vi "Actor Core.vi"(8 "error in":errorcluster, 11 "CS++DIM-Server in":refnum<class "CS++DIM-Server.lvclass">) -> (0 "error out":errorcluster, 3 "Actor out":refnum<class "Actor.lvclass">)   [LabVIEW 2015, in "CS++DIM-Server.lvlib" / "CS++DIM-Server.lvclass"]
doc: "(<B>Filename</B>: Actor Framework.lvlib:Actor.lvclass:Actor Core.vi)\n\nReceives messages to the actor, reacts to them, and initiates any error handling that may shut the actor down.\n\nDescendant classes may override this VI to append parallel tasks for the actor to complete while it handles messages. Overrides use the Call Parent Method node."
uses:
  CS++DIM-Server.lvclass
  <vilib>/ActorFramework/Actor/Actor.lvclass
  CSPP_Core/Actors/CS++BaseActor/CS++BaseActor.lvclass/CS++BaseActor.ctl
  CS++DIM-Server.lvclass/CS++DIM-Server.ctl
  <vilib>/ActorFramework/Actor/Actor.lvclass/Actor.ctl
  <vilib>/ActorFramework/Message Enqueuer/Message Enqueuer.lvclass/Message Enqueuer.ctl
  <vilib>/ActorFramework/Message Enqueuer/Init from Existing Queue.vi
  <vilib>/ActorFramework/Message Enqueuer/Enqueue.vi
  <vilib>/ActorFramework/Message Priority Queue/Priority Enqueue.vi
  <vilib>/ActorFramework/Stop Msg/Stop Msg.lvclass
  <vilib>/ActorFramework/Message Enqueuer/Message Enqueuer.lvclass
  CSPP_Core/Actors/CS++BaseActor/CS++BaseActor.lvclass
panel:
  out "Chart":dbl(graph)
  out "Update Rate":dbl[unit]
  out "Last Update":timestamp
  in  "Stop Button":bool
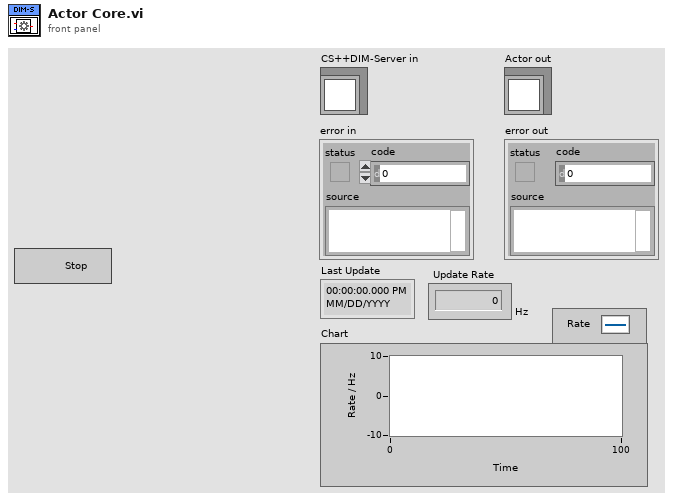
[diagram p1: front panel]
types:
  T1 = enum32{"Invalid", "Standard", "Closed", "Hidden", "Minimized", "Maximized"}
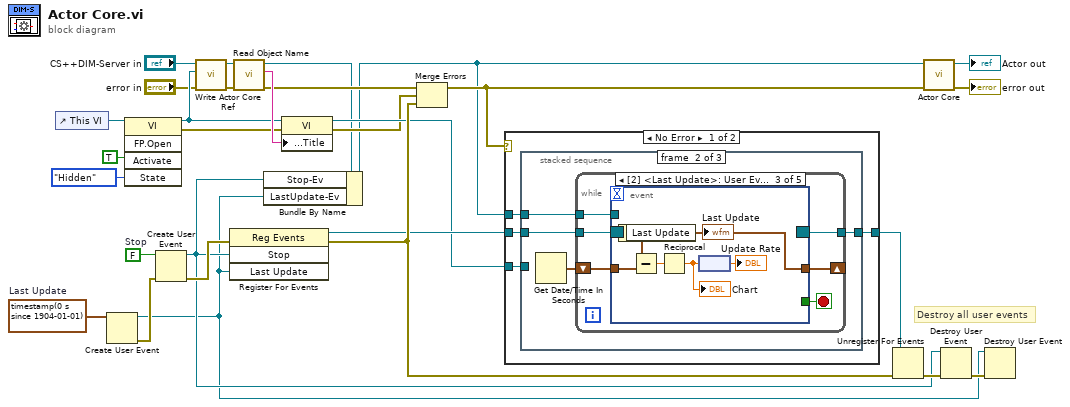
[diagram p0: block diagram]
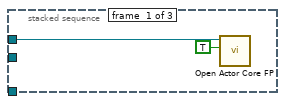
[diagram p2: hidden frame]
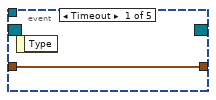
[diagram p3: hidden frame]
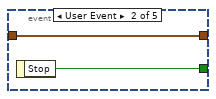
[diagram p4: hidden frame]
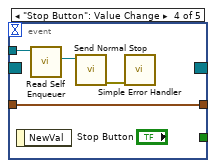
[diagram p5: hidden frame]
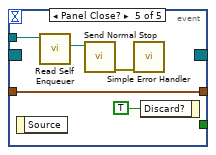
[diagram p6: hidden frame]
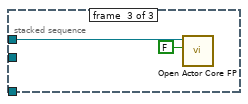
[diagram p7: hidden frame]
diagram:
  w7 = timestamp(0 s since 1904-01-01)  # Last Update
  w21 = FALSE  # Stop
  # "Destroy all user events"
  n1 = control-ref of="This VI"() -> (w25:refnum<vi>)
  n2 = Create User Event(user event datatype=w7) -> (user event=w1:refnum<user-event>, error out=w6:errorcluster)  [unwired: 1 in]
  n3 = invoke class="VI" method="FP.Open"(reference=w25, "Activate"=TRUE ("Activate?"), "State"=T1."Hidden") -> (reference out=w14:refnum<vi>, error out=w18:errorcluster)  [unwired: 2 in, 3 out]
  n4 = Create User Event(user event datatype=w21, error in=w6) -> (user event=w5:refnum<user-event>, error out=w19:errorcluster)
  n5 = call "Write Actor Core Ref.vi"("error in (no error)"="error in", "Actor Core Ref"=w14, "CS++BaseActor in"="CS++DIM-Server in") -> ("error out"=w17:errorcluster, "CS++BaseActor out"=w16:refnum<class "CS++DIM-Server.lvclass">)  [unwired: 7 in]
  n6 = register-events(error in=w19, w5, w1) -> (reference out=w28:refnum<event-registration>, error out=w29:errorcluster)  [unwired: 1 in]
  n7 = call "Read Object Name.vi"("error in (no error)"=w17, "CS++BaseActor in"=w16) -> ("error out"=w15:errorcluster, "Object Name"=w22:string, "CS++BaseActor out"=w4:refnum<class "CS++DIM-Server.lvclass">)  [unwired: 7 in]
  n8 = Bundle By Name(cluster=w4, "Stop-Ev"=w5, "LastUpdate-Ev"=w1) -> (w3:refnum<class "CS++DIM-Server.lvclass">)
  n9 = property class="VI"(reference=w14, error in=w18, "Front Panel.Title"=w22) -> (reference out=w27:refnum<vi>, error out=w20:errorcluster)
  n10 = Merge Errors(w15, w20, w29) -> (w26:errorcluster)
  n11 = case shown="No Error" w26 {
    tunnel: w3 -> [w33 _]
    tunnel: w28 -> [w32 w65]
    tunnel: [w31 w65] -> w10
    tunnel: w27 -> [w30 _]
    frame No Error {
      n12 = stacked-sequence {
        tunnel: w33 -> [w35 w38 w64]
        tunnel: w32 -> [_ w39 _]
        tunnel: [_ w37 _] -> w31
        tunnel: w30 -> [_ _ _]
        frame #0 {
          n13 = call "Open Actor Core FP.vi"("Open FP (F)"=TRUE, "CS++BaseActor in"=w35) -> ()  [unwired: 8 in, 2 out]
        }
        frame #1 {
          n14 = Get Date/Time In Seconds() -> (seconds since 1Jan1904=w36:timestamp)
          n15 = while {
            tunnel: w39 -> [w45]
            tunnel: w38 -> [w44]
            tunnel: [w42] -> w37
            shift-right: [w40] -> _
            shift-left: w36 -> [w41]
            stop <- w43 stop-if-true
            n16 = event shown="[2] <Last Update>: User Event" {
              selector: w45 -> [_ _ _ _ _]
              dyn-events: [_ _ _ _ _] -> w42
              timeout: _ -> [_ _ _ _ _]
              tunnel: w44 -> [_ _ _ w57 w59]
              tunnel: [_ w48 _ _ _] -> w43
              tunnel: w41 -> [w46 w47 w52 w54 w58]
              tunnel: [w46 w47 w53 w54 w58] -> w40
              event Timeout {
                n17 = event-data() -> ()  [unwired: 1 in, 1 out]
              }
              event User Event {
                n18 = event-data() -> ("Stop"=w48:bool)  [unwired: 1 in]
              }
              event User Event {
                n19 = event-data() -> ("Last Update"=w53:timestamp)  [unwired: 1 in]
                "Last Update" <- w53
                n20 = Subtract(x=w53, y=w52) -> (x-y=w51:dbl)
                n21 = Reciprocal(x=w51) -> (1/x=w49:dbl)
                "Chart" <- w49
                n22 = node(w49) -> (→"Update Rate":dbl[unit])
              }
              event "Stop Button": Value Change {
                n23 = event-data() -> ()  [unwired: 1 in, 1 out]
                n24 = call <vilib>:"Read Self Enqueuer.vi"("Actor"=w57) -> ("Self Enqueuer"=w56:refnum<class "Message Enqueuer.lvclass">)  [unwired: 10 in]
                n25 = call <vilib>:"Send Normal Stop.vi"("Message Enqueuer"=w56) -> ("error out"=w55:errorcluster)  [unwired: 10 in]
                n26 = call <vilib>:"Simple Error Handler.vi"("error in (no error)"=w55) -> ()  [unwired: 4 in, 5 out]
              }
              event Panel Close? {
                n27 = event-data() -> ()  [unwired: 1 in, 1 out]
                n28 = call <vilib>:"Read Self Enqueuer.vi"("Actor"=w59) -> ("Self Enqueuer"=w61:refnum<class "Message Enqueuer.lvclass">)  [unwired: 10 in]
                n29 = call <vilib>:"Send Normal Stop.vi"("Message Enqueuer"=w61) -> ("error out"=w60:errorcluster)  [unwired: 10 in]
                n30 = call <vilib>:"Simple Error Handler.vi"("error in (no error)"=w60) -> ()  [unwired: 4 in, 5 out]
                n31 = event-data("Discard?"=TRUE) -> ()  [unwired: 1 in, 1 out]
              }
            }
          }
        }
        frame #2 {
          n32 = call "Open Actor Core FP.vi"("Open FP (F)"=FALSE, "CS++BaseActor in"=w64) -> ()  [unwired: 8 in, 2 out]
        }
      }
    }
    frame Error {
    }
  }
  n33 = Unregister For Events(event registration refnum=w10, error in=w29) -> (error out=w11:errorcluster)
  n34 = call-parent "Actor Core.vi"("error in"=w26, "CS++BaseActor in"=w3) -> ("error out"=→"error out":errorcluster, "Actor out"=→"Actor out":refnum<class "Actor.lvclass">)  [unwired: 8 in]
  n35 = Destroy User Event(user event=w5, error in=w11) -> (error out=w2:errorcluster)
  n36 = Destroy User Event(user event=w1, error in=w2) -> ()  [unwired: 1 out]
